vi "Main.vi"() -> ()   [LabVIEW 2014]
uses:
  Klasy/Swiat/Swiat.lvclass
  Klasy/Swiat/Swiat.lvclass/Swiat.ctl
panel:
  in  "Stop":bool
  out "Swiat":picture caption="Œwiat"
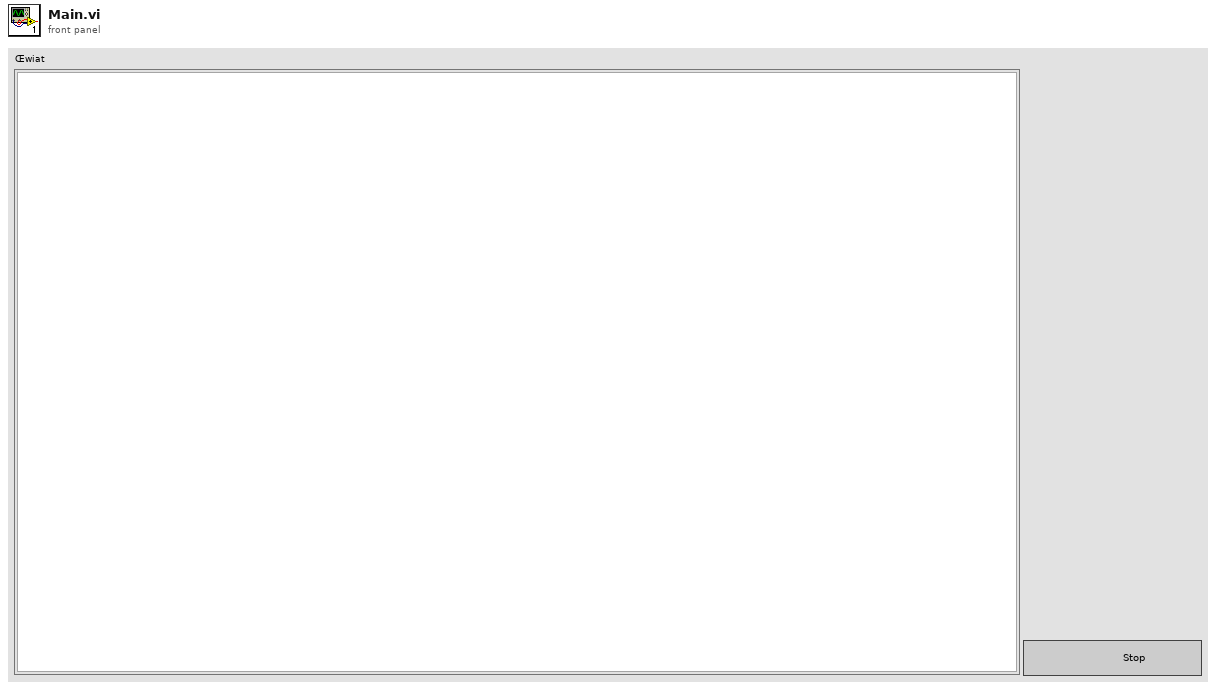
[diagram p1: front panel]
types:
  T1 = typedef "LVBoundsTypeDef.ctl" = cluster{"Width":u32, "Height":u32}
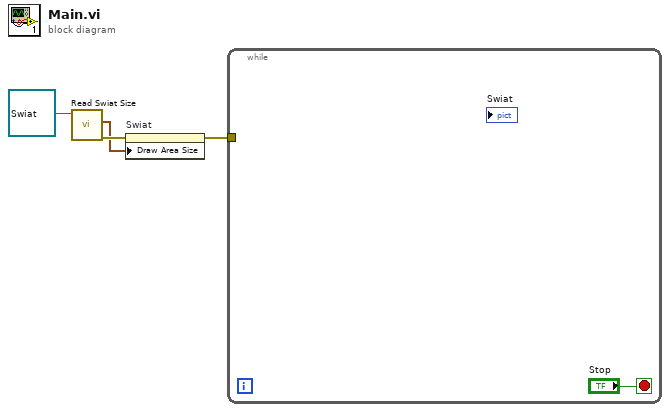
[diagram p0: block diagram]
diagram:
  n1 = call "Read Swiat Size.vi"("Swiat in"=refnum<class "Swiat.lvclass"> refnum ("Swiat.lvclass")) -> ("error out"=w3:errorcluster, "Size out"=w2:T1)  [unwired: 8 in, 1 out]
  n2 = property on="Swiat" class="Pict"(error in=w3, "Draw Area Size"=w2) -> (error out=w1:errorcluster)  [unwired: 1 in, 1 out]
  n3 = while {
    tunnel: w1 -> [_]
    stop <- "Stop" stop-if-true
  }
